vi "Delete Empty Folders.vi"(8 "error in (no error)":errorcluster, 11 "Rename in":refnum<class "ProjectItem.lvclass">) -> (0 "error out":errorcluster, 3 "Rename out":refnum<class "ProjectItem.lvclass">)   [LabVIEW 2019, in "ProjectItem.lvclass"]
uses:
  ProjectItem.lvclass
  ProjectItem.lvclass/ProjectItem.ctl
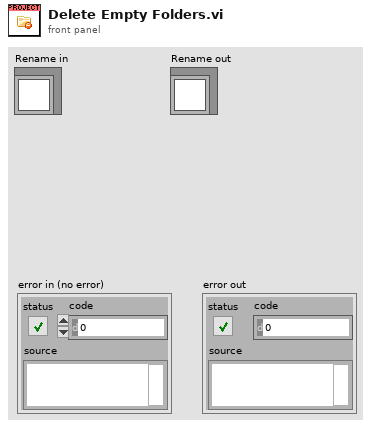
[diagram p1: front panel]
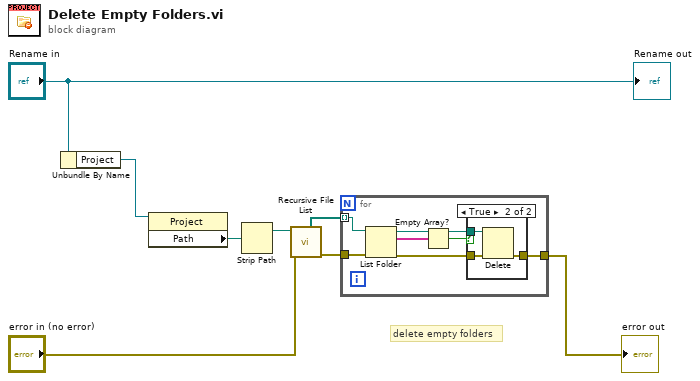
[diagram p0: block diagram]
diagram:
  # "delete empty folders"
  n1 = Unbundle By Name("Rename in") -> ("Project"=w8:refnum<vi>)
  n2 = property class="Project"(reference=w8) -> ("Path"=w3:path)  [unwired: 1 in, 2 out]
  n3 = Strip Path(path=w3) -> (stripped path=w4:path)  [unwired: 1 out]
  n4 = call <vilib>:"Recursive File List.vi"("error in (no error)"="error in (no error)", "Folder Path"=w4) -> ("error out"=w5:errorcluster, "All Folders"=w7:path[])  [unwired: 5 in, 3 out]
  n5 = for {
    tunnel: w5 -> [w15]
    tunnel: [w11] -> w6
    tunnel: w7 -> [w10] mode=indexing
    n6 = List Folder(path=w10, error in=w15) -> (path out=w13:path, filenames=w14:string[], error out=w12:errorcluster)  [unwired: 2 in, 1 out]
    n7 = Empty Array?(array=w14) -> (empty?=w9:bool)
    n8 = case shown="True" w9 {
      tunnel: w13 -> [_ w19]
      tunnel: w12 -> [w16 w18]
      tunnel: [w16 w17] -> w11
      frame False {
      }
      frame True {
        n9 = Delete(path (use dialog)=w19, error in=w18) -> (error out=w17:errorcluster)  [unwired: 3 in, 2 out]
      }
    }
  }
  "error out" <- w6
  "Rename out" <- "Rename in"
